vi "4bitFA.vi"(4 "Cin":bool, 6 "A1":bool, 7 "A2":bool, 8 "A4":bool, 9 "A8":bool) -> (0 "B2":bool, 1 "B4":bool, 2 "B8":bool, 3 "B1":bool, 5 "Cout":bool)   [LabVIEW 2018]
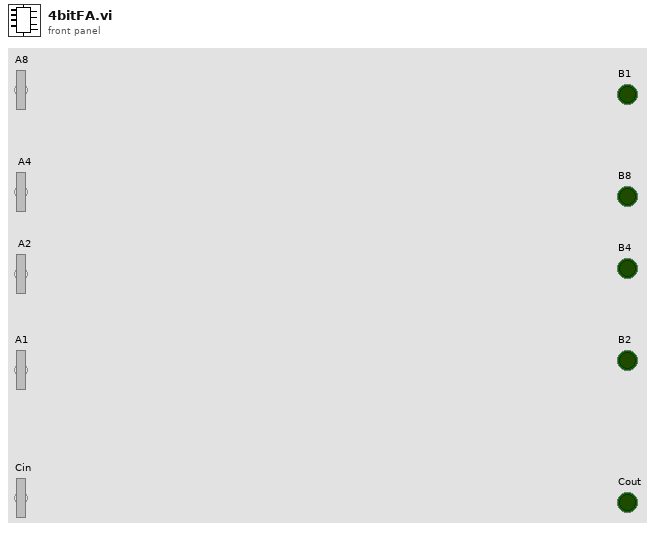
[diagram p1: front panel]
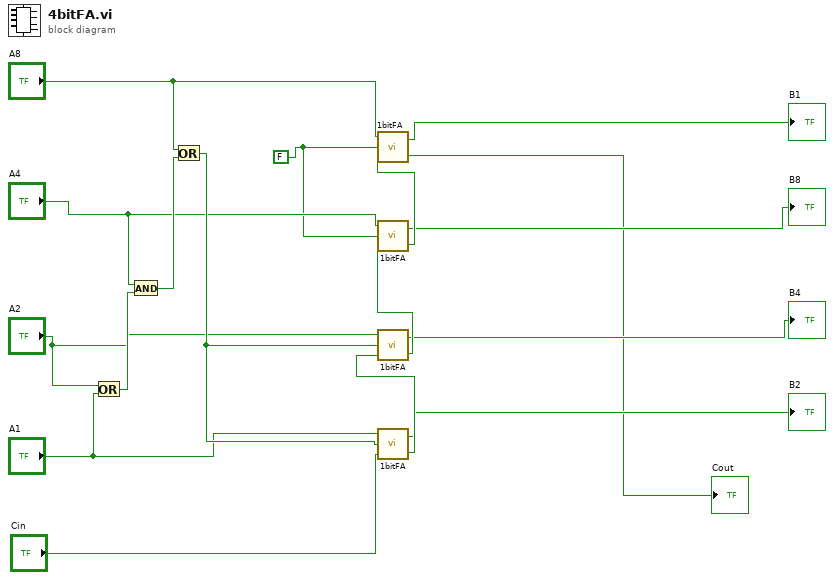
[diagram p0: block diagram]
diagram:
  w6 = FALSE
  n1 = Or(x="A2", y="A1") -> (x .or. y?=w17:bool)
  n2 = And(x="A4", y=w17) -> (x .and. y?=w16:bool)
  n3 = Or(x="A8", y=w16) -> (x .or. y?=w15:bool)
  n4 = call "1bitFA.vi"("Cin"="Cin", "B"=w15, "A"="A1") -> ("Cout"=w9:bool, "S"=→"B2":bool)
  n5 = call "1bitFA.vi"("Cin"=w9, "B"=w15, "A"="A2") -> ("Cout"=w8:bool, "S"=→"B4":bool)
  n6 = call "1bitFA.vi"("Cin"=w8, "B"=w6, "A"="A4") -> ("Cout"=w7:bool, "S"=→"B8":bool)
  n7 = call "1bitFA.vi"("Cin"=w7, "B"=w6, "A"="A8") -> ("Cout"=→"Cout":bool, "S"=→"B1":bool)
